vi "Evaluate Part 1.vi"() -> ()   [LabVIEW 2020]
uses:
  Proto/Proto.lvclass
panel:
  out "number":u64
  out "Array":bool[](array[boolean])
  in  "Input":string="x00: 1\nx01: 0\nx02: 1\nx03: 1\nx04: 0\ny00: 1\ny01: 1\ny02: 1\ny03: 1\ny04: 1\n\nntg XOR fgs -> mjb\ny02 OR x01 -> tnw\nkwq OR kpj -> z05\nx00 OR x03 -> fst\ntgd XOR rvg -> z01\nvdt OR tnw -> bfw\nbfw AND frj -> z10\nffh OR nrd -> bqk\ny00 AND y03 -> djm\ny03 OR y00 -> psh\nbqk OR frj -> z08\ntnw OR fst -> frj\ngnj AND tgd -> z11\nbfw XOR mjb -> z00\nx03 OR x00 -> vdt\ngnj AND wpb -> z02\nx04 AND y00 -> kjc\ndjm OR pbm -> qhw\nnrd AND vdt -> hwm\nkjc AND fst -> rvg\ny04 OR y02 -> fgs\ny01 AND x02 -> pbm\nntg OR kjc -> kwq\npsh XOR fgs -> tgd\nqhw XOR tgd -> z09\npbm OR djm -> kpj\nx03 XOR y03 -> ffh\nx00 XOR y04 -> ntg\nbfw OR bqk -> z06\nnrd XOR fgs -> wpb\nfrj XOR qhw -> z04\nbqk OR frj -> z07\ny03 OR x01 -> nrd\nhwm AND bqk -> z03\ntgd XOR rvg -> z12\ntnw OR pbm -> gnj"
  # "2947015374 too low\n\n282578783305985 too high\n66055249060558"
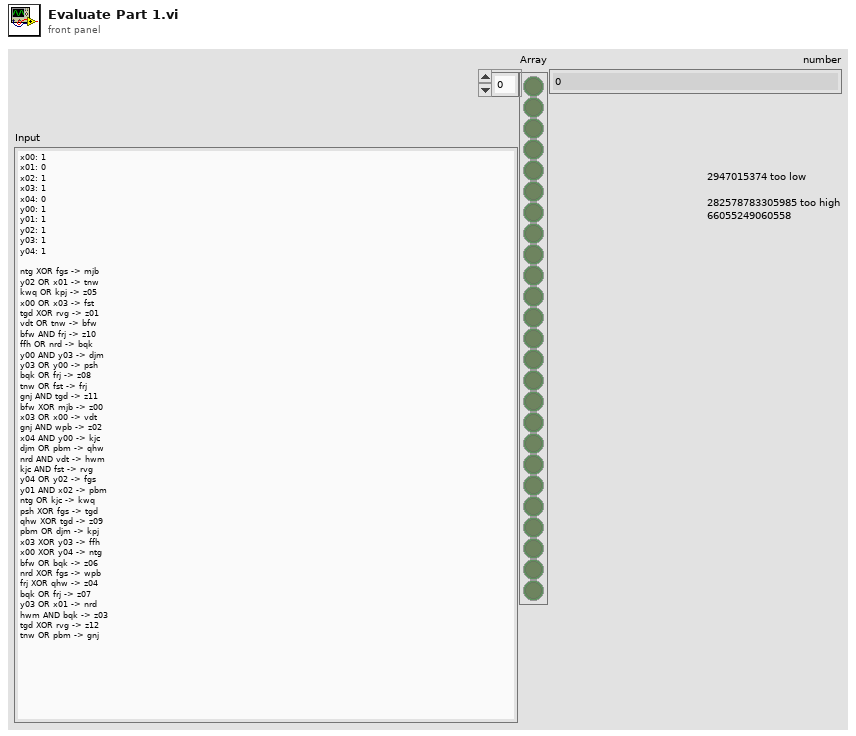
[diagram p1: front panel]
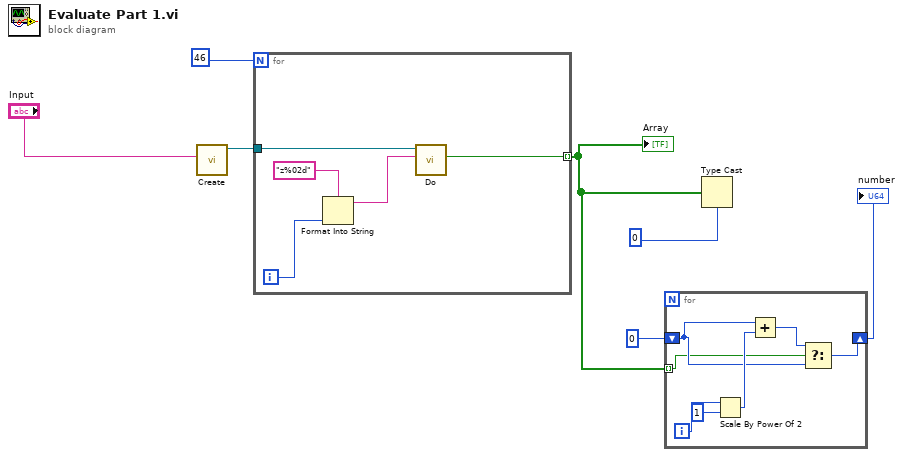
[diagram p0: block diagram]
diagram:
  n1 = call "Create.vi"("Input"="Input") -> ("Proto"=w7:refnum<class "Proto.lvclass">)  [unwired: 9 in, 1 out]
  n2 = for {
    N: 46 -> [_]
    tunnel: w7 -> [w12]
    tunnel: [w8] -> w4 mode=indexing
    i -> [w10]
    n3 = Format Into String(format string="z%02d", w10) -> (resulting string=w9:string)  [unwired: 2 in, 1 out]
    n4 = call "Do.vi"("Key"=w9, "Proto in"=w12) -> ("Value"=w8:bool)  [unwired: 7 in, 2 out]
  }
  "Array" <- w4
  n5 = for {
    tunnel: w4 -> [w15] mode=indexing
    shift-right: [w13] -> w2
    shift-left: u64 0 ("number") -> [w16]
    i -> [w19]
    n6 = Scale By Power Of 2(n=w19, x=u64 1) -> (x*2^n=w17:u64)
    n7 = Add(x=w16, y=w17) -> (x+y=w14:u64)
    n8 = Select(t=w14, s=w15, f=w16) -> (s? t:f=w13:u64)
  }
  "number" <- w2
  n9 = Type Cast(type=u64 0 ("number"), x=w4) -> ()  [unwired: 1 out]
